vi "Hide Splash.vi"(8 "error in (no error)":errorcluster, 11 "Plugin Splash in":refnum<class "Plugin Splash.lvclass">) -> (0 "error out":errorcluster, 3 "Plugin Splash out":refnum<class "Plugin Splash.lvclass">)   [LabVIEW 2020, in "Volatus.lvlib" / "Plugin Splash.lvclass"]
uses:
  Plugin Splash.lvclass
  Plugin Splash.lvclass/Plugin Splash.ctl
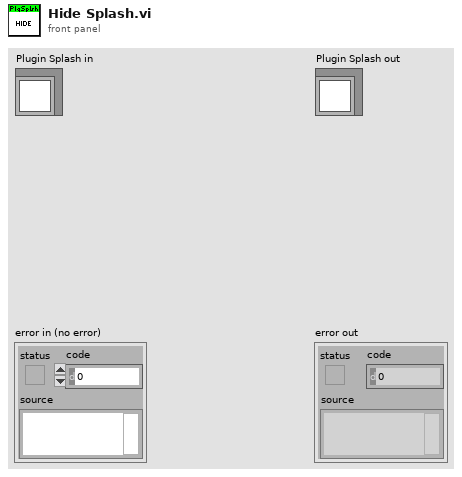
[diagram p1: front panel]
types:
  T1 = enum32{"Invalid", "Standard", "Closed", "Hidden", "Minimized", "Maximized"}
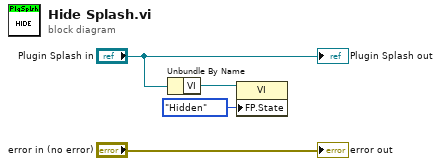
[diagram p0: block diagram]
diagram:
  n1 = Unbundle By Name("Plugin Splash in") -> ("VI"=w2:refnum<vi>)
  n2 = property class="VI"(reference=w2, "FP.State"=T1."Hidden" ("Front Panel Window:State")) -> ()  [unwired: 1 in, 2 out]
  "error out" <- "error in (no error)"
  "Plugin Splash out" <- "Plugin Splash in"
